vi "6733_write_waveform_standalone.vi"(11 "Inputs":T1 {"Waveform Parameters"."Degree" min=1}) -> (0 "error out":errorcluster, 2 "counter task":refnum<k21>, 3 "waveform task":refnum<k21>, 8 "error in (no error)":errorcluster)   [LabVIEW 2013]
uses:
  RydbergExpControl/red_mot_controls.ctl
  Control 1.ctl
  <vilib>/DAQmx/write.llb/DAQmx Write (Analog 1D DBL NChan 1Samp).vi
  <vilib>/DAQmx/write.llb/DAQmx Write (Analog 1D Wfm NChan NSamp).vi
  <vilib>/DAQmx/create/channels.llb/DAQmx Create Channel (AO-Voltage-Basic).vi
  <vilib>/DAQmx/miscellaneous.llb/DAQmx Fill In Error Info.vi
  <vilib>/Waveform/WDTOps.llb/WDT Append Waveforms DBL.vi
  <vilib>/DAQmx/configure/timing.llb/DAQmx Timing (Sample Clock).vi
  <vilib>/DAQmx/create/channels.llb/DAQmx Create Channel (CO-Pulse Generation-Frequency).vi
  <vilib>/DAQmx/configure/timing.llb/DAQmx Timing (Implicit).vi
  <vilib>/DAQmx/configure/trigger.llb/DAQmx Start Trigger (Digital Edge).vi
  <vilib>/Waveform/WDTOps.llb/WDT Scale Delta t DBL.vi
  <resource>/objmgr/daqmx.rc
panel:
  out "FIFO Buffer Size":dbl=16384.0
  in  "Stop":bool
  out "Total Time":dbl
  out "Sample Rate":dbl
  out "element":waveform(dbl)(graph)
  in  "index":i32
  out "Waveforms":waveform(dbl)[](array[waveform])
  out "Max Sample Rate":dbl=1000000.0
  out "# Inactive Channels":i32
  out "# Active Channels":i16
  out "Inactive Channels":tag[](array[tag])
  out "Active Channels":tag[](array[tag])
  out "Samples Written":dbl
  out "Voltage Maximum":dbl
  out "Voltage Minimum":dbl
  out "AO.PhysicalChans":tag[](array[tag])
  out "Active Device":tag
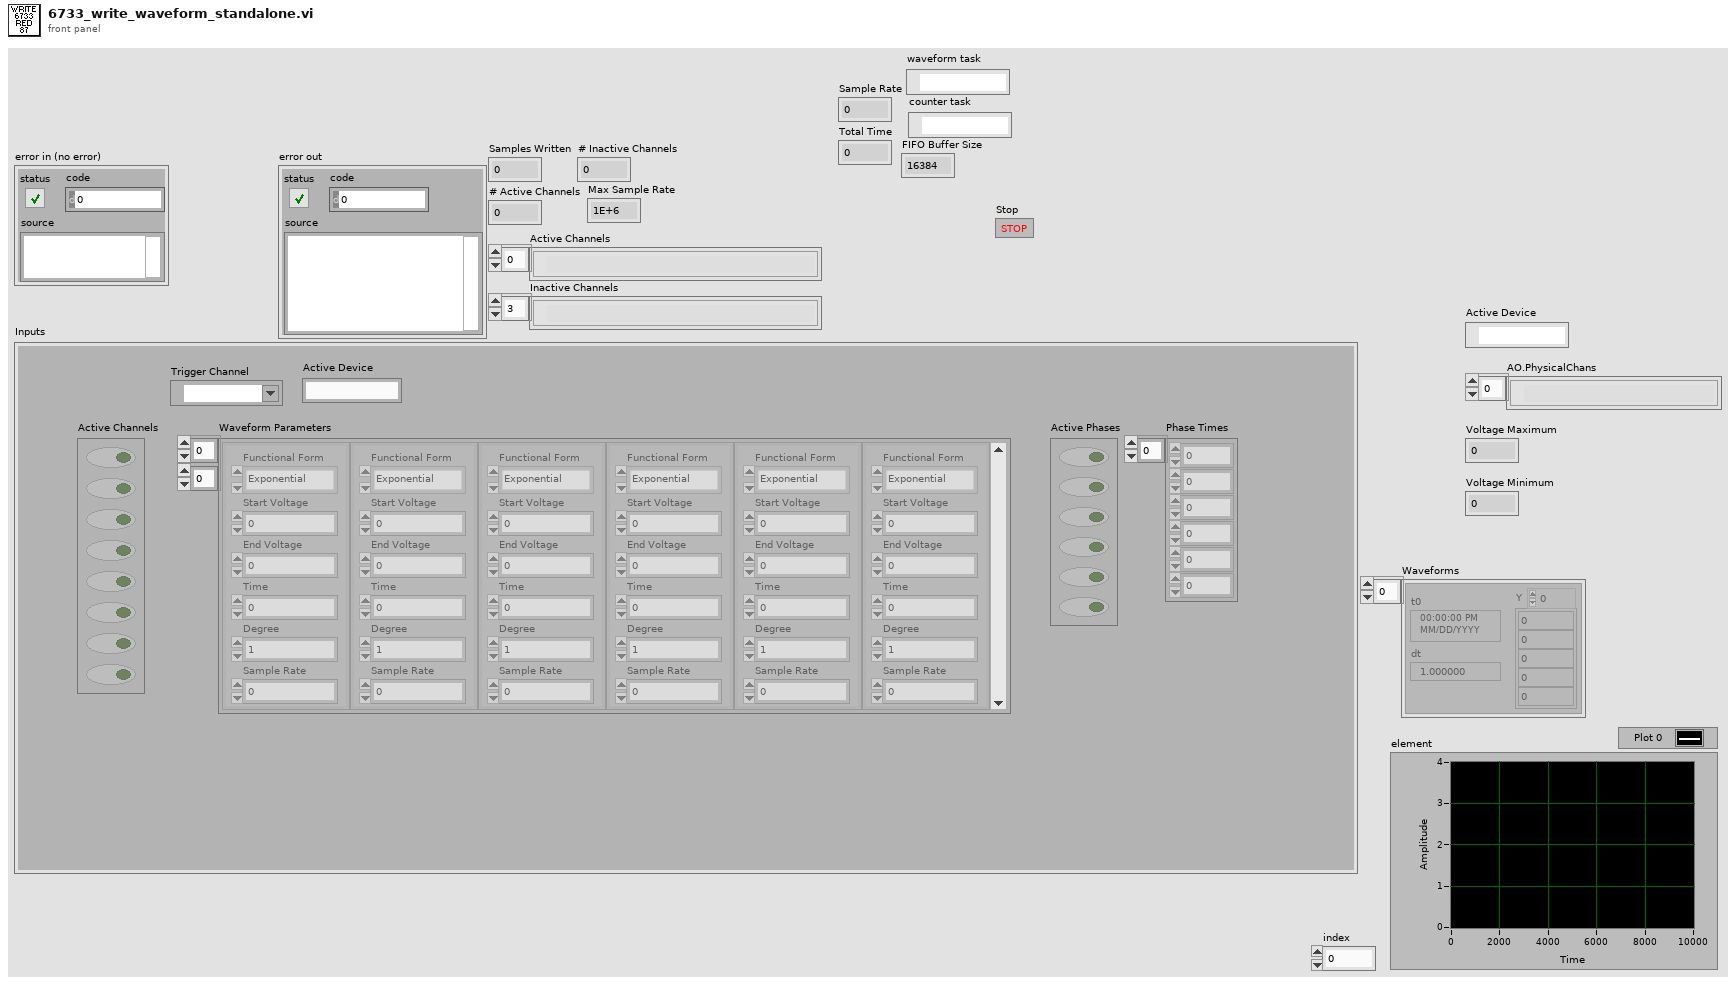
[diagram p1: front panel]
types:
  T1 = typedef "red_mot_controls.ctl" = cluster{"Active Device":string, "Active Channels":bool[], "Waveform Parameters":cluster{"Functional Form":enum16{"Polynomial", "Exponential"}, "Start Voltage":dbl, "End Voltage":dbl, "Time":dbl, "Degree":i8, "Sample Rate":dbl}[][], "Active Phases":bool[], "Phase Times":dbl[], "Trigger Channel":tag}
  T2 = typedef "Control 1.ctl" = enum16{"Initialize", "Get Device Information", "Get Active/Inactive Channels", "Maximize Samples / Channel", "Write Waveforms", "Check for Problems", "Clear Old Tasks", "Write to cards"}
  T3 = cluster{"Functional Form":enum16{"Polynomial", "Exponential"}, "Start Voltage":dbl, "End Voltage":dbl, "Time":dbl, "Degree":i8, "Sample Rate":dbl}[][]
  T4 = cluster{"Functional Form":enum16{"Polynomial", "Exponential"}, "Start Voltage":dbl, "End Voltage":dbl, "Time":dbl, "Degree":i8, "Sample Rate":dbl}[]
  T5 = cluster{"Functional Form":enum16{"Polynomial", "Exponential"}, "Start Voltage":dbl, "End Voltage":dbl, "Time":dbl, "Degree":i8, "Sample Rate":dbl}
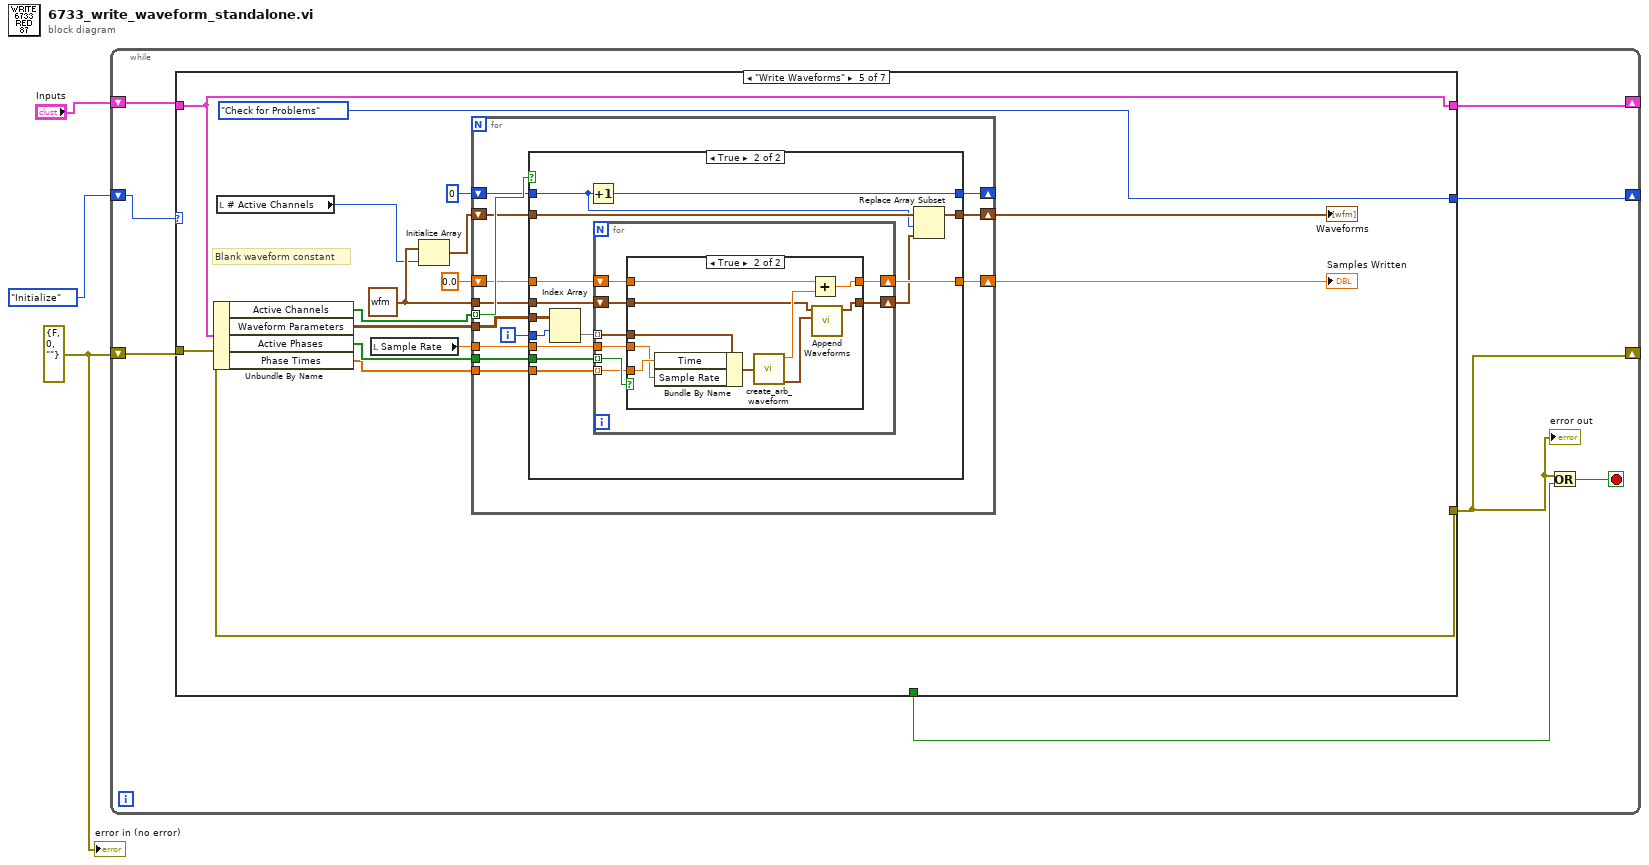
[diagram p0: block diagram]
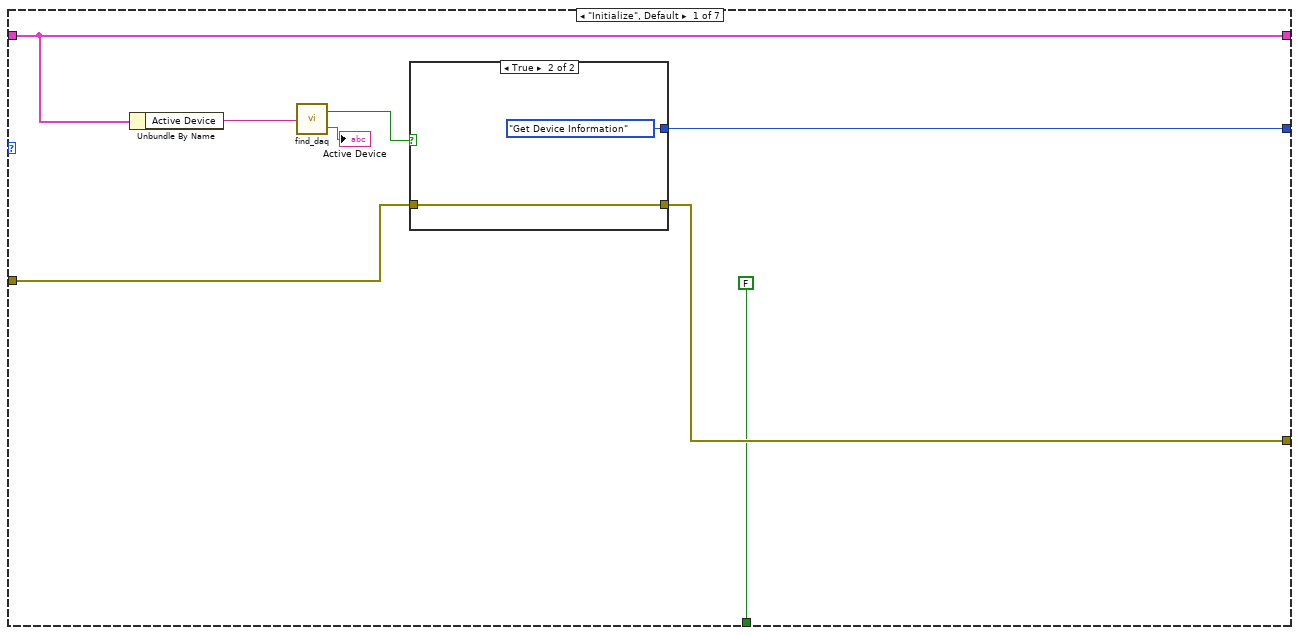
[diagram p2: hidden frame]
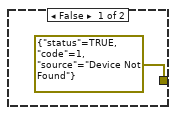
[diagram p3: hidden frame]
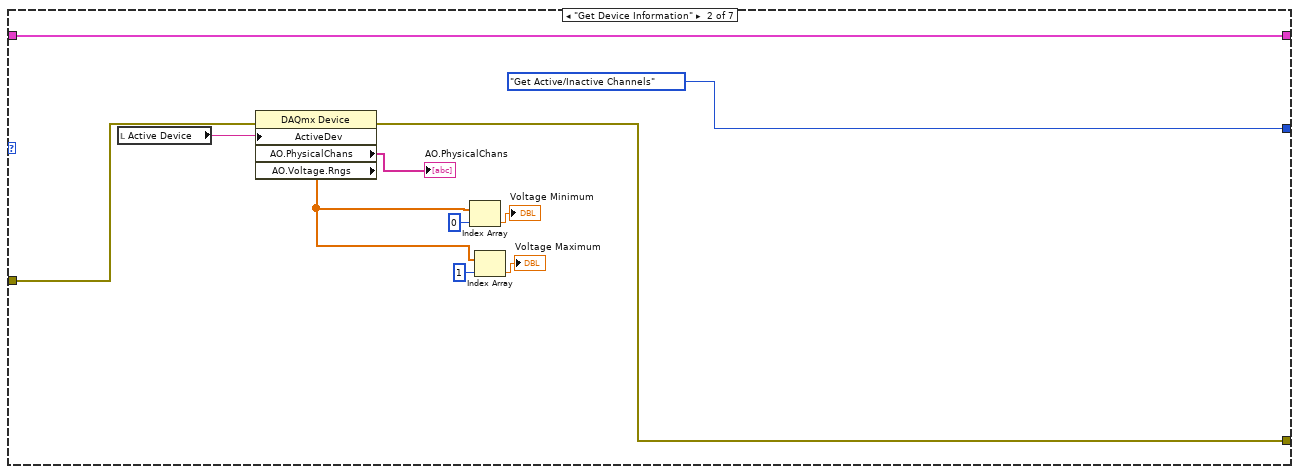
[diagram p4: hidden frame]
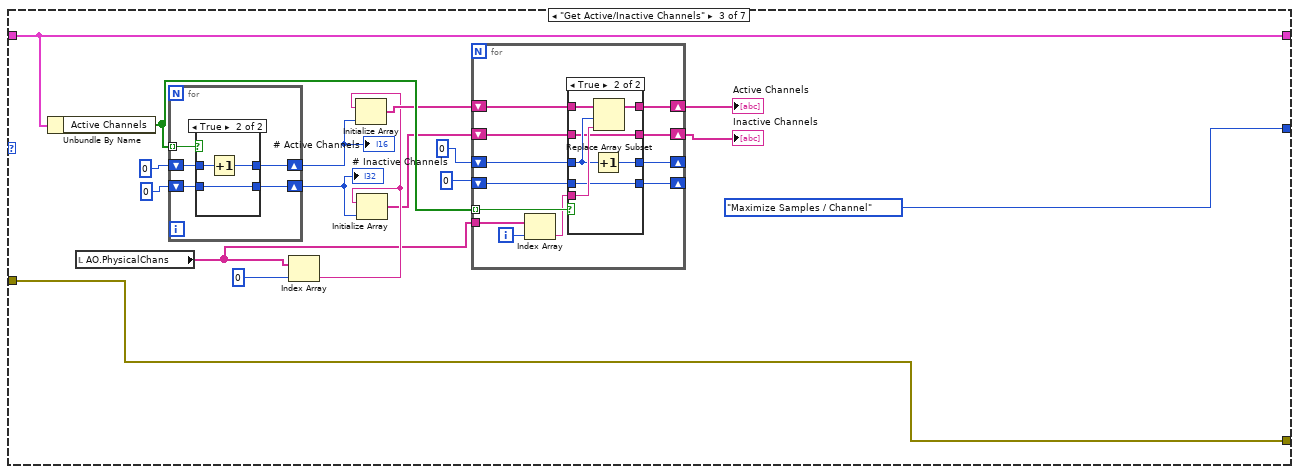
[diagram p5: hidden frame]
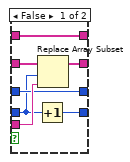
[diagram p6: hidden frame]
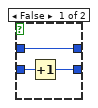
[diagram p7: hidden frame]
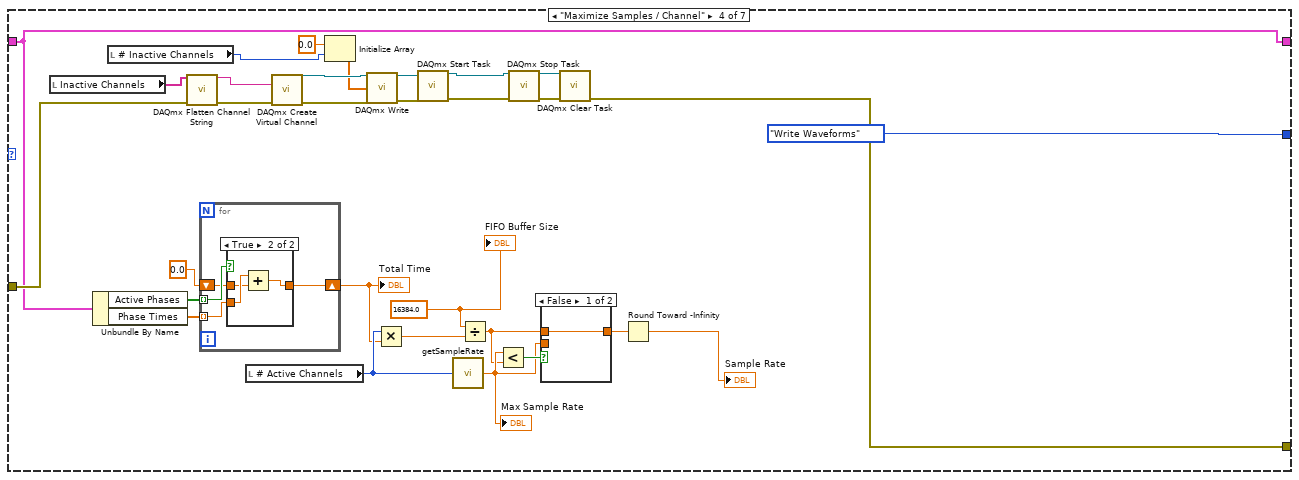
[diagram p8: hidden frame]
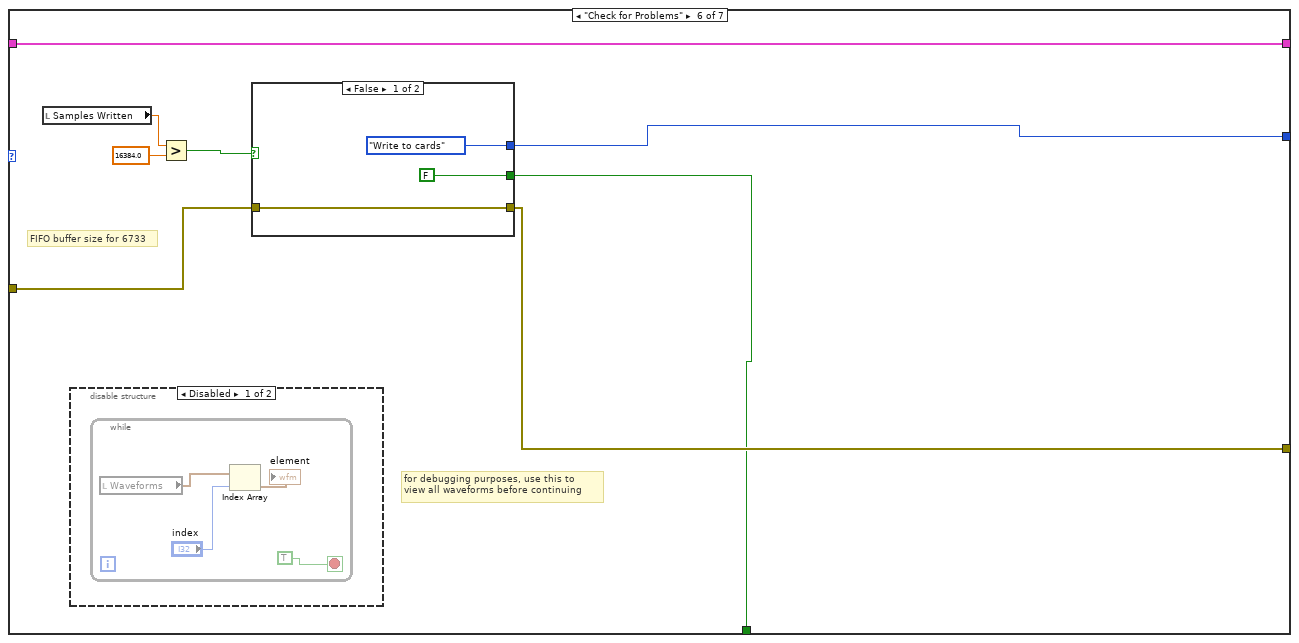
[diagram p13: hidden frame]
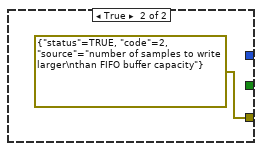
[diagram p15: hidden frame]
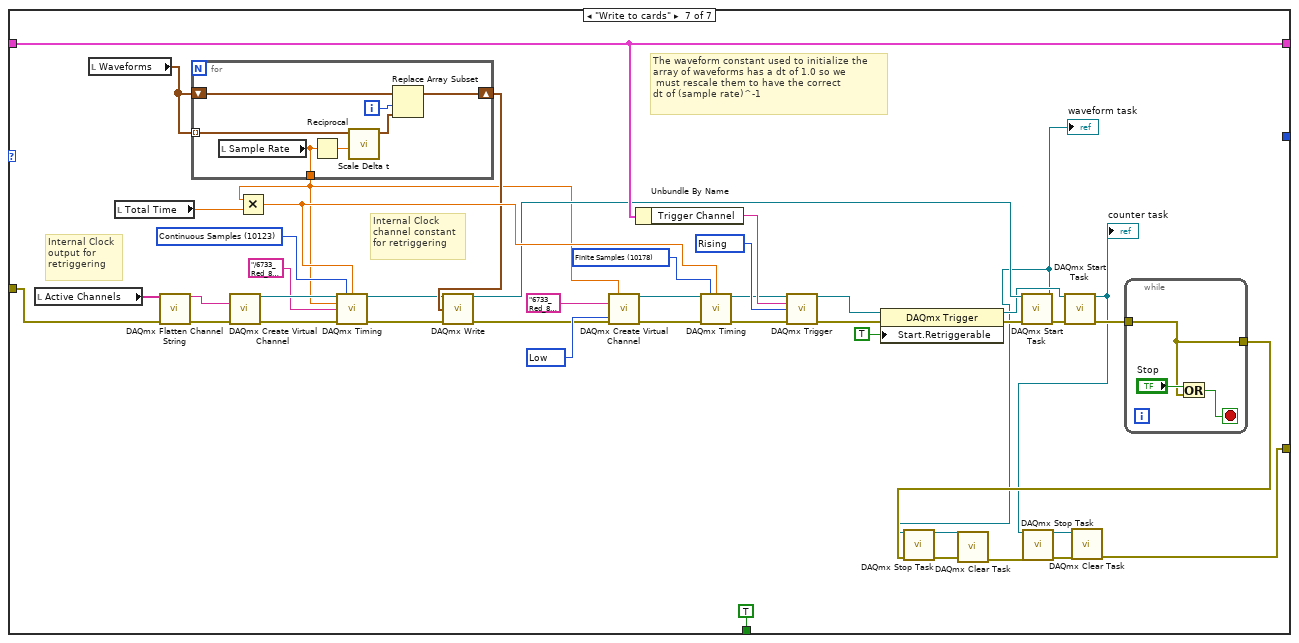
[diagram p16: hidden frame]
diagram:
  w1 = errorcluster {"status"=FALSE, "code"=0, "source"=""} ("error in (no error)")
  n1 = while {
    shift-right: [w4] -> _
    shift-left: w1 -> [w9]
    shift-right: [w8] -> _
    shift-left: Control_1."Initialize" -> [w11]
    shift-right: [w6] -> _
    shift-left: "Inputs" -> [w10]
    stop <- w7 stop-if-true
    n2 = case shown="\"Write Waveforms\"" w11 {
      tunnel: w10 -> [w13 w33 w37 w100 w138 w195 w250]
      tunnel: [w16 w24 w48 w104 w141 w196 w209] -> w4
      tunnel: w9 -> [w15 w32 w48 w115 w141 w197 w249]
      tunnel: [w14 Control_1."Get Active/Inactive Channels" Control_1."Maximize Samples / Channel" Control_1."Write Waveforms" Control_1."Check for Problems" w194 _] -> w8
      tunnel: [w13 w33 w37 w100 w138 w195 w250] -> w6
      tunnel: [FALSE ("y") _ _ _ _ w193 TRUE ("y")] -> w5
      frame "Initialize", Default {
        n3 = Unbundle By Name(w13) -> ("Active Device"=w19:string)
        n4 = call "find_daq.vi"("Device Name"=w19) -> ("Device Present"=w17:bool, "DAQmx Device Name"=→"Active Device":tag)
        n5 = case shown="True" w17 {
          tunnel: [errorcluster {"status"=TRUE, "code"=1, "source"="Device Not Found"} ("error in (no error)") w22] -> w16
          tunnel: w15 -> [_ w22]
          tunnel: [_ Control_1."Get Device Information"] -> w14
          frame False {
          }
          frame True {
          }
        }
      }
      frame "Get Device Information" {
        n6 = local read "Active Device"() -> (w31:tag)
        n7 = property class="DAQmx Device"(error in=w32, "ActiveDev"=w31) -> (error out=w24:errorcluster, "AO.PhysicalChans"=→"AO.PhysicalChans":tag[], "AO.Voltage.Rngs"=w26:dbl[])  [unwired: 1 in, 1 out]
        n8 = Index Array(array=w26, index=0) -> (element=→"Voltage Minimum":dbl)
        n9 = Index Array(array=w26, index=1) -> (element=→"Voltage Maximum":dbl)
      }
      frame "Get Active/Inactive Channels" {
        n10 = Unbundle By Name(w37) -> ("Active Channels"=w47:bool[])
        n11 = local read "AO.PhysicalChans"() -> (w41:tag[])
        n12 = for {
          shift-right: [w81] -> w46
          shift-left: i16 0 -> [w80]
          shift-right: [w79] -> w45
          shift-left: 0 -> [w78]
          tunnel: w47 -> [w77] mode=indexing
          n13 = case shown="True" w77 {
            tunnel: [w82 w87] -> w81
            tunnel: w80 -> [w82 w86]
            tunnel: [w84 w85] -> w79
            tunnel: w78 -> [w83 w85]
            frame False {
              n14 = Increment(x=w83) -> (x+1=w84:i32)
            }
            frame True {
              n15 = Increment(x=w86) -> (x+1=w87:i16)
            }
          }
        }
        "# Active Channels" <- w46
        "# Inactive Channels" <- w45
        n16 = Index Array(array=w41, index=0) -> (element=w42:tag)
        n17 = Initialize Array(w42, w46) -> (w44:tag[])
        n18 = Initialize Array(w42, w45) -> (w40:tag[])
        n19 = for {
          tunnel: w47 -> [w62] mode=indexing
          shift-right: [w59] -> w36
          shift-left: w44 -> [w60]
          tunnel: w41 -> [w57]
          shift-right: [w55] -> w35
          shift-left: w40 -> [w56]
          shift-right: [w53] -> _
          shift-left: 0 ("index") -> [w54]
          shift-right: [w51] -> _
          shift-left: 0 ("index") -> [w52]
          i -> [w61]
          n20 = Index Array(array=w57, index=w61) -> (element=w58:tag)
          n21 = case shown="True" w62 {
            tunnel: w60 -> [w63 w76]
            tunnel: [w63 w75] -> w59
            tunnel: w58 -> [w69 w74]
            tunnel: w56 -> [w68 w70]
            tunnel: [w67 w70] -> w55
            tunnel: w54 -> [w66 w73]
            tunnel: [w66 w72] -> w53
            tunnel: w52 -> [w65 w71]
            tunnel: [w64 w71] -> w51
            frame False {
              n22 = Increment(x=w65) -> (x+1=w64:i32)
              n23 = Replace Array Subset(array=w68, new element=w69, index=w65) -> (w67:tag[])
            }
            frame True {
              n24 = Increment(x=w73) -> (x+1=w72:i32)
              n25 = Replace Array Subset(array=w76, new element=w74, index=w73) -> (w75:tag[])
            }
          }
        }
        "Active Channels" <- w36
        "Inactive Channels" <- w35
      }
      frame "Maximize Samples / Channel" {
        w96 = 16384.0
        n26 = local read "Inactive Channels"() -> (w116:tag[])
        n27 = Unbundle By Name(w100) -> ("Active Phases"=w99:bool[], "Phase Times"=w98:dbl[])
        n28 = local read "# Inactive Channels"() -> (w109:i32)
        n29 = call <vilib>:"DAQmx Flatten Channel String.vi"("names in"=w116, "error in"=w115) -> ("names out"=w114:string, "error out"=w117:errorcluster)  [unwired: 12 in]
        n30 = for {
          tunnel: w99 -> [w123] mode=indexing
          tunnel: w98 -> [w122] mode=indexing
          shift-right: [w120] -> w88
          shift-left: 0.0 -> [w121]
          n31 = case shown="True" w123 {
            tunnel: w122 -> [_ w127]
            tunnel: w121 -> [w124 w126]
            tunnel: [w124 w125] -> w120
            frame False {
            }
            frame True {
              n32 = Add(x=w127, y=w126) -> (x+y=w125:dbl)
            }
          }
        }
        "Total Time" <- w88
        n33 = local read "# Active Channels"() -> (w89:i16)
        n34 = call-poly <vilib>:"DAQmx Create Virtual Channel.vi"("physical channels"=w114, "error in"=w117) -> ("task out"=w113:refnum<k21>, "error out"=w112:errorcluster)  [unwired: 12 in]
        n35 = Initialize Array(0.0 ("element"), w109) -> (w107:dbl[])
        n36 = call-poly <vilib>:"DAQmx Write.vi"("task/channels in"=w113, "data"=w107, "error in"=w112) -> ("task out"=w110:refnum<k21>, "error out"=w111:errorcluster)  [unwired: 10 in, 1 out]
        n37 = Multiply(x=w89, y=w88) -> (x*y=w90:dbl)
        n38 = call <vilib>:"DAQmx Start Task.vi"("task/channels in"=w110, "error in"=w111) -> ("task out"=w102:refnum<k21>, "error out"=w103:errorcluster)  [unwired: 12 in]
        n39 = call "getSampleRate.vi"("Number of active channels"=w89) -> ("Sample Rate"=w94:dbl)
        "Max Sample Rate" <- w94
        n40 = Divide(x=w96, y=w90) -> (x/y=w93:dbl)
        n41 = Less?(x=w94, y=w93) -> (x < y?=w95:bool)
        n42 = call <vilib>:"DAQmx Stop Task.vi"("task/channels in"=w102, "error in"=w103) -> ("task out"=w106:refnum<k21>, "error out"=w105:errorcluster)  [unwired: 12 in]
        n43 = case shown="False" w95 {
          tunnel: [w118 w119] -> w92
          tunnel: w94 -> [_ w119]
          tunnel: w93 -> [w118 _]
          frame False {
          }
          frame True {
          }
        }
        n44 = call <vilib>:"DAQmx Clear Task.vi"("task in"=w106, "error in"=w105) -> ("error out"=w104:errorcluster)  [unwired: 13 in]
        n45 = Round Toward -Infinity(1:w92) -> (0:→"Sample Rate":dbl)
        "FIFO Buffer Size" <- w96
      }
      frame "Write Waveforms" {
        w135 = waveform(dbl) {"t0"=timestamp(0 s since 1904-01-01), "dt"=1.0, "Y"=[]}
        # "Blank waveform constant"
        n46 = Unbundle By Name(w138) -> ("Active Channels"=w130:bool[], "Waveform Parameters"=w142:T3, "Active Phases"=w136:bool[], "Phase Times"=w131:dbl[])
        n47 = local read "# Active Channels"() -> (w128:i16)
        n48 = local read "Sample Rate"() -> (w129:dbl)
        n49 = Initialize Array(w135, w128) -> (w133:waveform(dbl)[])
        n50 = for {
          tunnel: w130 -> [w155] mode=indexing
          tunnel: w142 -> [w153]
          shift-right: [w152] -> w140
          shift-left: 0.0 -> [w151]
          tunnel: w136 -> [w150]
          tunnel: w135 -> [w149]
          shift-right: [w147] -> _
          shift-left: 0 -> [w148]
          shift-right: [w145] -> w132
          shift-left: w133 -> [w146]
          tunnel: w131 -> [w144]
          tunnel: w129 -> [w143]
          i -> [w154]
          n51 = case shown="True" w155 {
            tunnel: w154 -> [_ w172]
            tunnel: w153 -> [_ w171]
            tunnel: [w158 w170] -> w152
            tunnel: w151 -> [w158 w169]
            tunnel: w150 -> [_ w167]
            tunnel: w149 -> [_ w166]
            tunnel: w148 -> [w157 w163]
            tunnel: [w157 w165] -> w147
            tunnel: w146 -> [w156 w164]
            tunnel: [w156 w161] -> w145
            tunnel: w144 -> [_ w160]
            tunnel: w143 -> [_ w159]
            frame False {
            }
            frame True {
              n52 = Index Array(array=w171, index (row)=w172) -> (element=w168:T4)  [unwired: 1 in]
              n53 = Increment(x=w163) -> (x+1=w165:i32)
              n54 = for {
                shift-right: [w180] -> w170
                shift-left: w169 -> [w179]
                tunnel: w168 -> [w178] mode=indexing
                shift-right: [w176] -> w162
                shift-left: w166 -> [w177]
                tunnel: w167 -> [w175] mode=indexing
                tunnel: w160 -> [w174] mode=indexing
                tunnel: w159 -> [w173]
                n55 = case shown="True" w175 {
                  tunnel: [w182 w191] -> w180
                  tunnel: w179 -> [w182 w190]
                  tunnel: w178 -> [_ w186]
                  tunnel: w177 -> [w181 w188]
                  tunnel: [w181 w187] -> w176
                  tunnel: w174 -> [_ w185]
                  tunnel: w173 -> [_ w183]
                  frame False {
                  }
                  frame True {
                    n56 = Bundle By Name(cluster=w186, "Time"=w185, "Sample Rate"=w183) -> (w184:T5)
                    n57 = call "create_arb_waveform.vi"("Waveform Parameters"=w184) -> ("Samples to Write"=w192:dbl, "output waveform"=w189:waveform(dbl))  [unwired: 2 out]
                    n58 = Add(x=w190, y=w192) -> (x+y=w191:dbl)
                    n59 = call-poly <vilib>:"Append Waveforms.vi"("waveform B"=w189, "waveform A"=w188) -> ("waveform out"=w187:waveform(dbl))  [unwired: 8 in, 1 out]
                  }
                }
              }
              n60 = Replace Array Subset(array=w164, new element=w162, index=w163) -> (w161:waveform(dbl)[])
            }
          }
        }
        "Samples Written" <- w140
        "Waveforms" <- w132
      }
      frame "Check for Problems" {
        # "FIFO buffer size for 6733"
        # "for debugging purposes, use this to\nview all waveforms before continuing"
        n61 = local read "Samples Written"() -> (w200:dbl)
        n62 = disable-structure shown="Disabled" {
          frame Disabled {
            n63 = while {
              stop <- TRUE stop-if-true
              n64 = local read "Waveforms"() -> (w204:waveform(dbl)[])
              n65 = Index Array(array=w204, index="index") -> (element=→"element":waveform(dbl))
            }
          }
          frame Enabled {
          }
        }
        n66 = Greater?(x=w200, y=16384.0) -> (0:w199:bool)
        n67 = case shown="False" w199 {
          tunnel: w197 -> [w207 _]
          tunnel: [w207 errorcluster {"status"=TRUE, "code"=2, "source"="number of samples to write larger\nthan FIFO buffer capacity"} ("error in (no error)")] -> w196
          tunnel: [Control_1."Write to cards" _] -> w194
          tunnel: [FALSE ("y") _] -> w193
          frame False {
          }
          frame True {
          }
        }
      }
      frame "Write to cards" {
        w231 = 10280 items=["Rising"=10280, "Falling"=10171] ("edge")
        w240 = 10123 items=["Finite Samples"=10178, "Continuous Samples"=10123, "Hardware Timed Single Point"=12522] ("sample mode")
        w242 = 10178 items=["Finite Samples"=10178, "Continuous Samples"=10123, "Hardware Timed Single Point"=12522] ("sample mode")
        w245 = 10214 items=["High"=10192, "Low"=10214] ("idle state")
        # "The waveform constant used to initialize the\narray of waveforms has a dt of 1.0 so we\n must rescale them to have the correct \ndt of (sample rate)^-1"
        # "Internal Clock\noutput for\nretriggering"
        # "Internal Clock\nchannel constant\nfor retriggering"
        n68 = local read "Active Channels"() -> (w247:tag[])
        n69 = local read "Waveforms"() -> (w251:waveform(dbl)[])
        n70 = local read "Total Time"() -> (w241:dbl)
        n71 = call <vilib>:"DAQmx Flatten Channel String.vi"("names in"=w247, "error in"=w249) -> ("names out"=w246:string, "error out"=w248:errorcluster)  [unwired: 12 in]
        n72 = for {
          tunnel: w251 -> [w262] mode=indexing
          shift-right: [w256] -> w235
          shift-left: w251 -> [w258]
          tunnel: [w257] -> w221
          i -> [w260]
          n73 = local read "Sample Rate"() -> (w257:dbl)
          n74 = Reciprocal(x=w257) -> (1/x=w261:dbl)
          n75 = call-poly <vilib>:"Scale Delta t.vi"("scale factor"=w261, "waveform in"=w262) -> ("waveform out"=w259:waveform(dbl))  [unwired: 8 in, 1 out]
          n76 = Replace Array Subset(array=w258, new element=w259, index=w260) -> (w256:waveform(dbl)[])
        }
        n77 = call-poly <vilib>:"DAQmx Create Virtual Channel.vi"("physical channels"=w246, "error in"=w248) -> ("task out"=w238:refnum<k21>, "error out"=w237:errorcluster)  [unwired: 12 in]
        n78 = Multiply(x=w221, y=w241) -> (x*y=w239:dbl)
        n79 = call-poly <vilib>:"DAQmx Timing.vi"("task/channels in"=w238, "sample mode"=w240, "samples per channel"=w239, "rate"=w221, "source"=tag "/6733_Red_87/Ctr0InternalOutput", "error in"=w237) -> ("task out"=w234:refnum<k21>, "error out"=w236:errorcluster)  [unwired: 8 in]
        n80 = call-poly <vilib>:"DAQmx Write.vi"("task/channels in"=w234, "data"=w235, "error in"=w236) -> ("task out"=w225:refnum<k21>, "error out"=w233:errorcluster)  [unwired: 10 in, 1 out]
        n81 = call-poly <vilib>:"DAQmx Create Virtual Channel.vi"("frequency"=w221, "counter"=tag "6733_Red_87/ctr0", "error in"=w233, "idle state"=w245) -> ("task out"=w244:refnum<k21>, "error out"=w243:errorcluster)  [unwired: 10 in]
        n82 = Unbundle By Name(w250) -> ("Trigger Channel"=w230:tag)
        n83 = call-poly <vilib>:"DAQmx Timing.vi"("task/channels in"=w244, "sample mode"=w242, "samples per channel"=w239, "error in"=w243) -> ("task out"=w229:refnum<k21>, "error out"=w232:errorcluster)  [unwired: 10 in]
        n84 = call-poly <vilib>:"DAQmx Trigger.vi"("task/channels in"=w229, "source"=w230, "edge"=w231, "error in"=w232) -> ("task out"=w227:refnum<k21>, "error out"=w228:errorcluster)  [unwired: 10 in]
        n85 = property class="DAQmx Trigger"(reference=w227, error in=w228, "Start.Retriggerable"=TRUE) -> (reference out=w222:refnum<k21>, error out=w224:errorcluster)
        n86 = call <vilib>:"DAQmx Start Task.vi"("task/channels in"=w225, "error in"=w224) -> ("task out"=w211:refnum<k21>, "error out"=w223:errorcluster)  [unwired: 12 in]
        "waveform task" <- w211
        n87 = call <vilib>:"DAQmx Start Task.vi"("task/channels in"=w222, "error in"=w223) -> ("task out"=w210:refnum<k21>, "error out"=w218:errorcluster)  [unwired: 12 in]
        "counter task" <- w210
        n88 = while {
          tunnel: w218 -> [w253]
          tunnel: [w253] -> w212
          stop <- w255 stop-if-true
          n89 = Or(x="Stop", y=w253) -> (x .or. y?=w255:bool)
        }
        n90 = call <vilib>:"DAQmx Stop Task.vi"("task/channels in"=w211, "error in"=w212) -> ("task out"=w217:refnum<k21>, "error out"=w216:errorcluster)  [unwired: 12 in]
        n91 = call <vilib>:"DAQmx Clear Task.vi"("task in"=w217, "error in"=w216) -> ("error out"=w215:errorcluster)  [unwired: 13 in]
        n92 = call <vilib>:"DAQmx Stop Task.vi"("task/channels in"=w210, "error in"=w215) -> ("task out"=w214:refnum<k21>, "error out"=w213:errorcluster)  [unwired: 12 in]
        n93 = call <vilib>:"DAQmx Clear Task.vi"("task in"=w214, "error in"=w213) -> ("error out"=w209:errorcluster)  [unwired: 13 in]
      }
    }
    "error out" <- w4
    n94 = Or(x=w4, y=w5) -> (x .or. y?=w7:bool)
  }
  "error in (no error)" <- w1
